vi "UpdateStimulusGivenTrack.vi"(8 "error in (no error)":errorcluster, 9 "CameraFrame":i32, 10 "Track":T1, 11 "StimulusObject in":refnum<class "StimulusObject.lvclass">) -> (0 "error out":errorcluster, 2 "StimulusObject Changed":bool, 3 "StimulusObject out":refnum<class "StimulusObject.lvclass">)   [LabVIEW 2019, in "StimulusObject.lvclass"]
uses:
  StimulusObject.lvclass
  WormTrackCluster.ctl
  TrackTerminationReasonEnum.ctl
  StimulusObject.lvclass/StimulusObject.ctl
  ParametersGlobal.vi
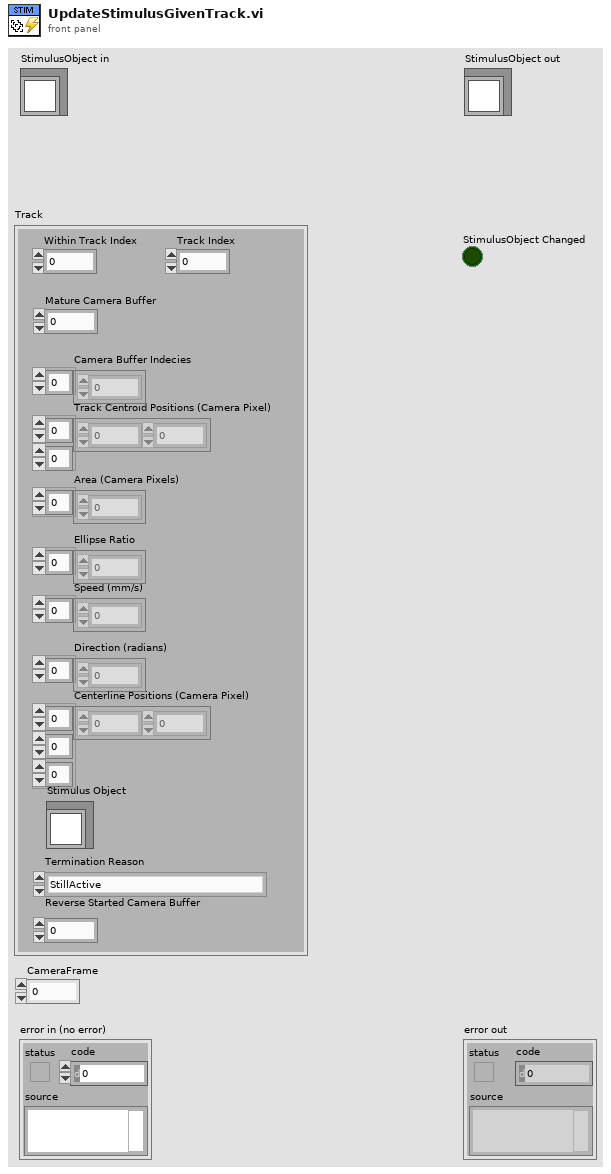
[diagram p1: front panel]
types:
  T1 = typedef "WormTrackCluster.ctl" = cluster{"Track Centroid Positions (Camera Pixel)":sgl[][], "Within Track Index":i32, "Camera Buffer Indecies":i32[], "Area (Camera Pixels)":i32[], "Speed (mm/s)":sgl[], "Direction (radians)":sgl[], "Centerline Positions (Camera Pixel)":sgl[][][], "Ellipse Ratio":sgl[], "Stimulus Object":refnum<class "StimulusObject.lvclass">, "Termination Reason":T2, "Track Index":i32, "Mature Camera Buffer":i32, "Reverse Started Camera Buffer":i32}
  T2 = typedef "TrackTerminationReasonEnum.ctl" = enum16{"StillActive", "MaxDisplacement", "NoBlobsLeft", "AreaIncrease", "AreaDecrease", "ExperimentEnded"}
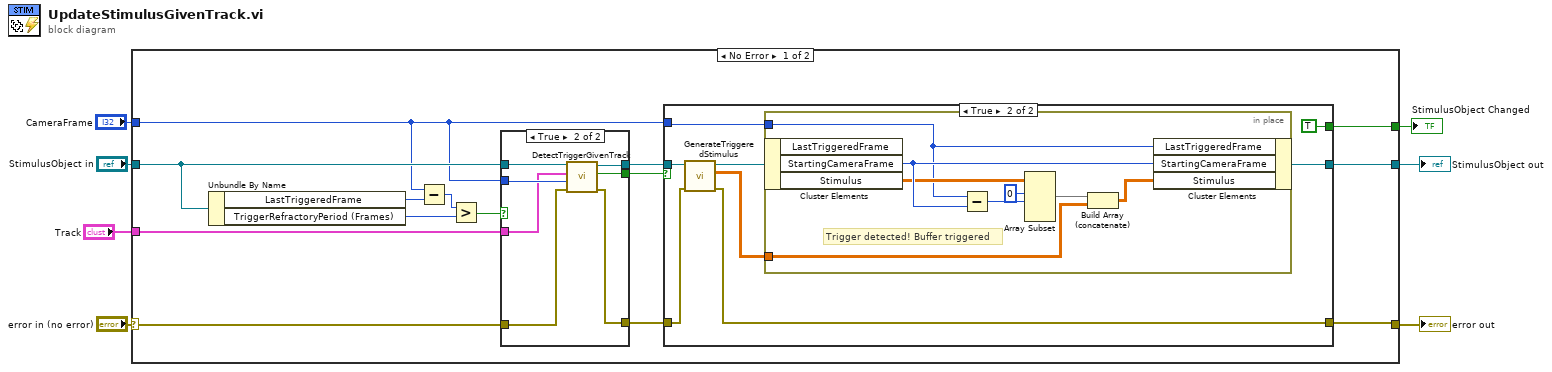
[diagram p0: block diagram]
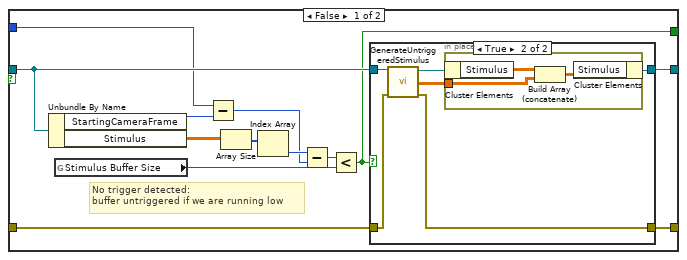
[diagram p2: hidden frame]
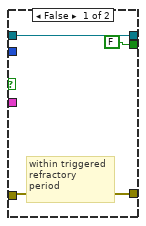
[diagram p4: hidden frame]
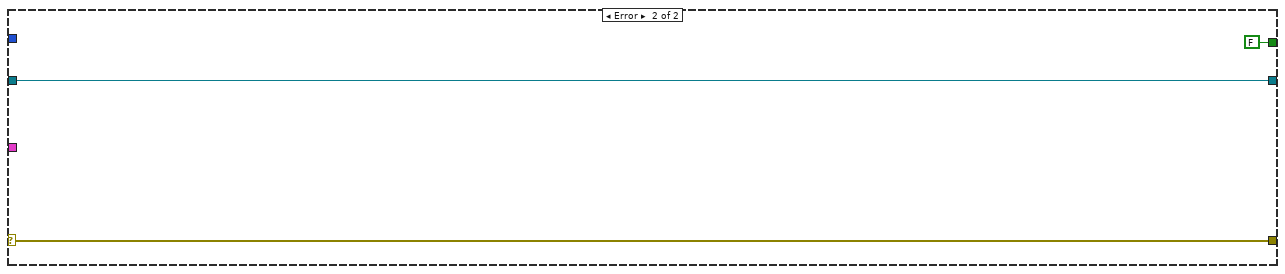
[diagram p5: hidden frame]
diagram:
  n1 = case shown="No Error" "error in (no error)" {
    selector: "error in (no error)" -> [w14 w74]
    tunnel: [w20 w74] -> w6
    tunnel: [w21 w73] -> w4
    tunnel: "StimulusObject in" -> [w17 w73]
    tunnel: "Track" -> [w10 _]
    tunnel: "CameraFrame" -> [w9 _]
    tunnel: [w8 FALSE] -> w1
    frame No Error {
      n2 = Unbundle By Name(w17) -> ("LastTriggeredFrame"=w19:i32, "TriggerRefractoryPeriod (Frames)"=w18:i32)
      n3 = Subtract(x=w9, y=w19) -> (x-y=w11:i32)
      n4 = Greater?(x=w11, y=w18) -> (0:w16:bool)
      n5 = case shown="True" w16 {
        tunnel: w17 -> [w64 w71]
        tunnel: [w64 w70] -> w15
        tunnel: w9 -> [_ w69]
        tunnel: w14 -> [w63 w68]
        tunnel: [w63 w67] -> w13
        tunnel: [FALSE ("Triggered?") w66] -> w12
        tunnel: w10 -> [_ w65]
        frame False {
          # "within triggered\nrefractory\nperiod"
        }
        frame True {
          n6 = call-dynamic "DetectTriggerGivenTrack.vi"("error in (no error)"=w68, "CameraFrame"=w69, "Track"=w65, "StimulusObject in"=w71) -> ("error out"=w67:errorcluster, "Triggered?"=w66:bool, "StimulusObject out"=w70:refnum<class "StimulusObject.lvclass">)  [unwired: 5 in]
        }
      }
      n7 = case shown="True" w12 {
        tunnel: [w33 w47] -> w21
        tunnel: [w32 w50] -> w20
        tunnel: w15 -> [w27 w53]
        tunnel: w13 -> [w26 w52]
        tunnel: w9 -> [w24 w49]
        tunnel: [w22 TRUE] -> w8
        frame False {
          # "No trigger detected:\nbuffer untriggered if we are running low"
          n8 = Unbundle By Name(w27) -> ("StartingCameraFrame"=w34:i32, "Stimulus"=w25:sgl[][])
          n9 = global read "ParametersGlobal.vi" "Stimulus Buffer Size"() -> (w23:i32)
          n10 = Subtract(x=w24, y=w34) -> (x-y=w28:i32)
          n11 = Array Size(array=w25) -> (size(s)=w31:i32[])
          n12 = Index Array(array=w31) -> (element=w29:i32)  [unwired: 1 in]
          n13 = Subtract(x=w29, y=w28) -> (x-y=w30:i32)
          n14 = Less?(x=w30, y=w23) -> (x < y?=w22:bool)
          n15 = case shown="True" w22 {
            tunnel: w27 -> [w36 w42]
            tunnel: [w36 w37] -> w33
            tunnel: w26 -> [w35 w41]
            tunnel: [w35 w40] -> w32
            frame False {
            }
            frame True {
              n16 = call-dynamic "GenerateUntriggeredStimulus.vi"("error in (no error)"=w41, "StimulusObject in"=w42) -> ("error out"=w40:errorcluster, "UntriggeredStimulusOut"=w38:sgl[][], "StimulusObject out"=w39:refnum<class "StimulusObject.lvclass">)  [unwired: 7 in]
              n17 = in-place {
                in-place-border: w38 -> [w43]
                n18 = in-place-cluster #1(w39) -> ("Stimulus"=w45:sgl[][])
                n19 = Build Array (concatenate)(w45, w43) -> (w44:sgl[][])
                n20 = in-place-cluster #1("Stimulus"=w44) -> (w37:refnum<class "StimulusObject.lvclass">)
              }
            }
          }
        }
        frame True {
          n21 = call-dynamic "GenerateTriggeredStimulus.vi"("error in (no error)"=w52, "Stimulus in"=w53) -> ("error out"=w50:errorcluster, "TriggeredStimulus"=w48:sgl[][], "Stimulus out"=w51:refnum<class "StimulusObject.lvclass">)  [unwired: 7 in]
          n22 = in-place {
            in-place-border: w49 -> [w55]
            in-place-border: w48 -> [w56]
            # "Trigger detected! Buffer triggered"
            n23 = in-place-cluster #2(w51) -> ("StartingCameraFrame"=w61:i32, "Stimulus"=w60:sgl[][])  [unwired: 1 out]
            n24 = Subtract(x=w55, y=w61) -> (x-y=w58:i32)
            n25 = Array Subset(array=w60, index (row)=0 ("index"), length (row)=w58) -> (w57:sgl[][])  [unwired: 2 in]
            n26 = Build Array (concatenate)(w57, w56) -> (w54:sgl[][])
            n27 = in-place-cluster #2("LastTriggeredFrame"=w55, "StartingCameraFrame"=w61, "Stimulus"=w54) -> (w47:refnum<class "StimulusObject.lvclass">)
          }
        }
      }
    }
    frame Error {
    }
  }
  "error out" <- w6
  "StimulusObject out" <- w4
  "StimulusObject Changed" <- w1
